vi "Improved Error Dialog.vi"(6 "Modal":bool=TRUE caption="Modal (T)", 8 "error in (no error)":errorcluster, 10 "Dialog Type":T1, 11 "Clear Error":bool caption="Clear Error (F)") -> (0 "error out":errorcluster)   [LabVIEW 2017, in "Error Dialog w Copy to Clipboard.lvlib"]
doc: "Displays a revamped error dialog to the user which improve the capabilities by offering to :\n- copy the error code & message into the clipboard.\n- open the search ni.com for the error code.\n- display either a dialog box with a single close window option (after the user acknowledges the dialog box, the VI returns control to the main VI) or a dialog box with buttons, which the user can use to either continue or stop (if the user selects Stop, the VI calls the Stop function to halt execution).\n\nBSD 3-Clause License\n\nCopyright (c) 2022, Neosoft Technologies Inc\nAll rights reserved.\n\nRedistribution and use in source and binary forms, with or without\nmodification, are permitted provided that the following conditions are met:\n\n1. Redistributions of source code must retain the above copyright notice, this\n list of conditions and the following disclaimer.\n\n2. Redistributions in binary form must reproduce the above copyright notice,\n this list of conditions and the following disclaimer in the documentation\n and/or other materials provided with the distribution.\n\n3. Neither the name of the copyright holder nor the names of its\n contributors may be used to endorse or promote products derived from\n this software without specific prior written permission.\n\nTHIS SOFTWARE IS PROVIDED BY THE COPYRIGHT HOLDERS AND CONTRIBUTORS \"AS IS\"\nAND ANY EXPRESS OR IMPLIED WARRANTIES, INCLUDING, BUT NOT LIMITED TO, THE\nIMPLIED WARRANTIES OF MERCHANTABILITY AND FITNESS FOR A PARTICULAR PURPOSE ARE\nDISCLAIMED. IN NO EVENT SHALL THE COPYRIGHT HOLDER OR CONTRIBUTORS BE LIABLE\nFOR ANY DIRECT, INDIRECT, INCIDENTAL, SPECIAL, EXEMPLARY, OR CONSEQUENTIAL\nDAMAGES (INCLUDING, BUT NOT LIMITED TO, PROCUREMENT OF SUBSTITUTE GOODS OR\nSERVICES; LOSS OF USE, DATA, OR PROFITS; OR BUSINESS INTERRUPTION) HOWEVER\nCAUSED AND ON ANY THEORY OF LIABILITY, WHETHER IN CONTRACT, STRICT LIABILITY,\nOR TORT (INCLUDING NEGLIGENCE OR OTHERWISE) ARISING IN ANY WAY OUT OF THE USE\nOF THIS SOFTWARE, EVEN IF ADVISED OF THE POSSIBILITY OF SUCH DAMAGE."
uses:
  Error Dialog w Copy to Clipboard.lvlib
  Dialog Type.ctl
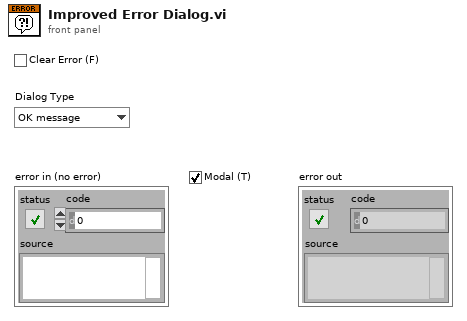
[diagram p1: front panel]
types:
  T1 = typedef "Error Dialog w Copy to Clipboard.lvlib/Dialog Type.ctl" = enum16{"OK message", "Continue or Stop message"}
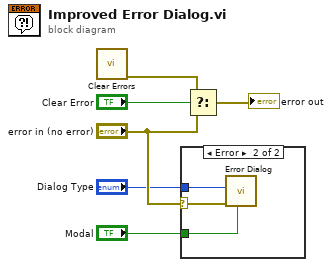
[diagram p0: block diagram]
diagram:
  n1 = call <vilib>:"Clear Errors.vi"() -> ("error out"=w3:errorcluster)  [unwired: 6 in, 1 out]
  n2 = case shown="Error" "error in (no error)" {
    selector: "error in (no error)" -> [_ w8]
    tunnel: "Modal" -> [_ w9]
    tunnel: "Dialog Type" -> [_ w7]
    frame No Error {
    }
    frame Error {
      n3 = call "Error Dialog.vi"("Modal (T)"=w9, "error in (no error)"=w8, "Dialog Type"=w7) -> ()  [unwired: 8 in, 1 out]
    }
  }
  n4 = Select(t=w3, s="Clear Error", f="error in (no error)") -> (s? t:f=→"error out":errorcluster)
